vi "Ignore 1073676294.vi"(8 "error in (no error)":errorcluster) -> (0 "error out":errorcluster)   [LabVIEW 2015, in "niDTS CommLib.lvlib" / "niDTS Comm Serial.lvclass"]
uses:
  niDTS Comm Serial.lvclass
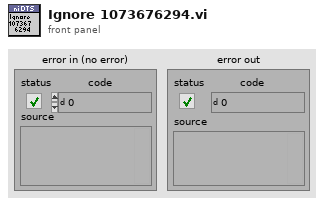
[diagram p1: front panel]
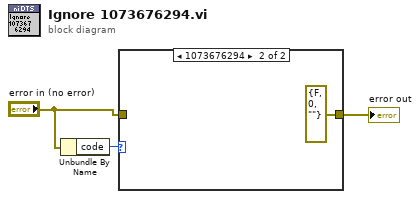
[diagram p0: block diagram]
diagram:
  n1 = Unbundle By Name("error in (no error)") -> ("code"=w1:i32)
  n2 = case shown="1073676294" w1 {
    tunnel: "error in (no error)" -> [w4 _]
    tunnel: [w4 errorcluster {"status"=FALSE, "code"=0, "source"=""} ("error in")] -> w2
    frame Default {
    }
    frame 1073676294 {
    }
  }
  "error out" <- w2
